vi "EMS CID File Error.vi"(8 "error in (no error)":errorcluster, 9 "Error Information":string, 10 "File Name":string, 11 "Master Controller in":refnum<class "Master Controller.lvclass">) -> (0 "error out":errorcluster, 3 "Master Controller out":refnum<class "Master Controller.lvclass">)   [LabVIEW 2015, in "Master Controller Core.lvlib" / "Master Controller.lvclass"]
uses:
  Master Controller.lvclass
  Communications/SCADA Communcations Actor/SCADA Communications/Controls/EMS Message Cluster.ctl
  Master Controller.lvclass/Master Controller.ctl
  Communications/SCADA Communcations Actor/SCADA Communications Messages/Transmit EMS Message Msg/Transmit EMS Message Msg.lvclass/Transmit EMS Message Msg.ctl
  <vilib>/ActorFramework/Message Enqueuer/Message Enqueuer.lvclass/Message Enqueuer.ctl
  <vilib>/ActorFramework/Message Enqueuer/Enqueue.vi
  <vilib>/ActorFramework/Message Priority Queue/Priority Enqueue.vi
  Communications/SCADA Communcations Actor/SCADA Communications Messages/Transmit EMS Message Msg/Transmit EMS Message Msg.lvclass
  Communications/SCADA Communcations Actor/SCADA Communications/SCADA Communications.lvclass
  Utilities/Message Strings.llb/Message String Utilities.lvlib
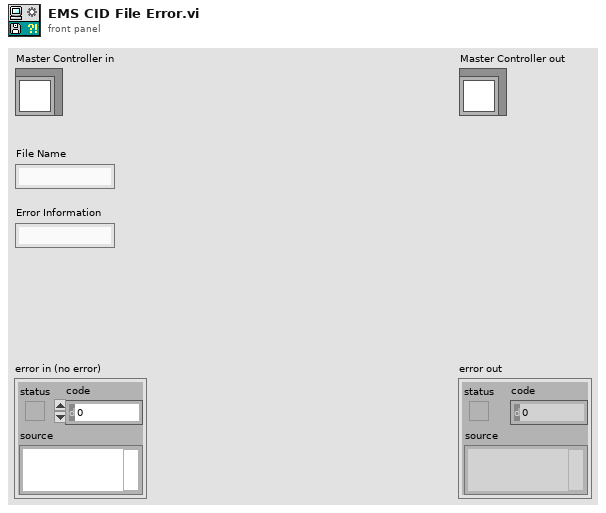
[diagram p1: front panel]
types:
  T1 = typedef "SCADA Communcations Actor.lvlib/SCADA Communications.lvclass/EMS Message Cluster.ctl" = cluster{"Name":string, "Content":string}
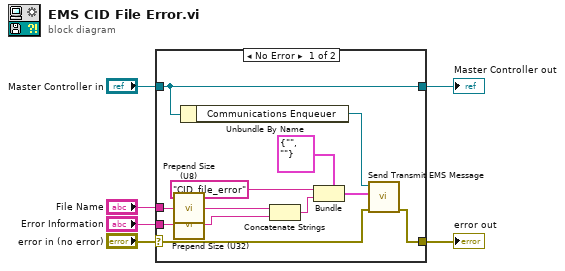
[diagram p0: block diagram]
diagram:
  n1 = case shown="No Error" "error in (no error)" {
    selector: "error in (no error)" -> [w12 w20]
    tunnel: [w13 w20] -> w5
    tunnel: [w18 w19] -> w3
    tunnel: "Master Controller in" -> [w18 w19]
    tunnel: "File Name" -> [w11 _]
    tunnel: "Error Information" -> [w10 _]
    frame No Error {
      n2 = call "Prepend Size (U8).vi"("String in"=w11) -> ("String out"=w9:string)
      n3 = call "Prepend Size (U32).vi"("String in"=w10) -> ("String out"=w8:string)
      n4 = Unbundle By Name(w18) -> ("Communications Enqueuer"=w17:refnum<class "Message Enqueuer.lvclass">)
      n5 = Concatenate Strings(w9, w8) -> (w15:string)
      n6 = Bundle(cluster=T1 {"Name"="", "Content"=""} ("Message"), "Name"="CID_file_error", "Content"=w15) -> (w14:T1)
      n7 = call "Send Transmit EMS Message.vi"("error in (no error)"=w12, "Message"=w14, "Message Enqueuer"=w17) -> ("error out"=w13:errorcluster)  [unwired: 7 in, 1 out]
    }
    frame Error {
    }
  }
  "error out" <- w5
  "Master Controller out" <- w3
